vi "Get Server DLL Path.vi"() -> (0 "server dll path":path)   [LabVIEW 2019, in "grpc-lvsupport.lvlib"]
uses:
  grpc-lvsupport.lvlib
  <vilib>/Utility/LVLibp/NI_PackedLibraryUtility.lvlib
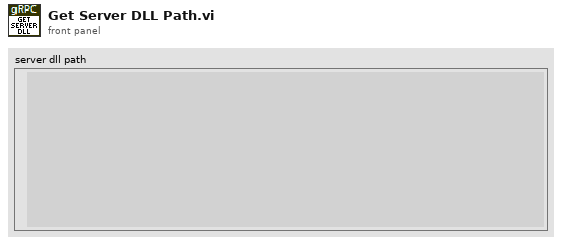
[diagram p1: front panel]
types:
  T1 = enum32{"invalid app kind", "Development System", "Run Time System", "Student Edition", "Embedded LabVIEW", "Evaluation", "Custom"}
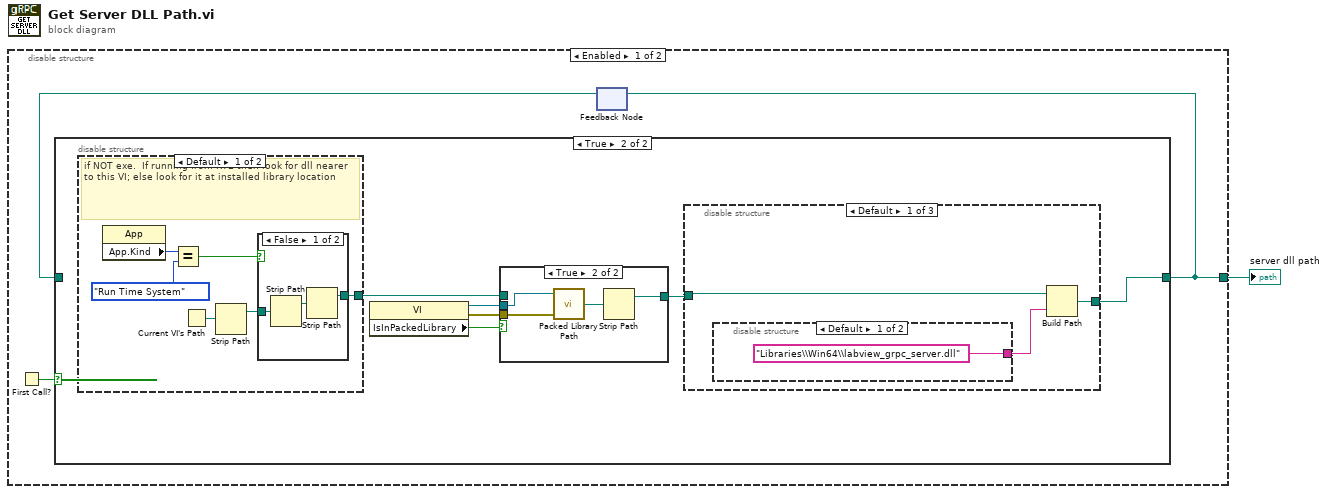
[diagram p0: block diagram]
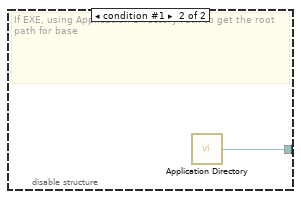
[diagram p5: hidden frame]
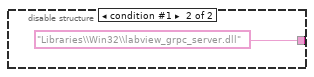
[diagram p6: hidden frame]
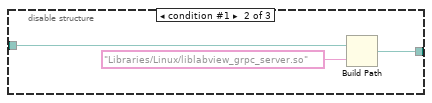
[diagram p7: hidden frame]
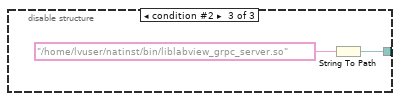
[diagram p8: hidden frame]
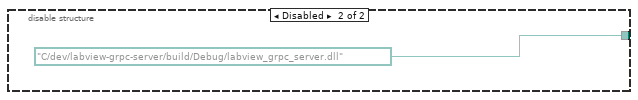
[diagram p9: hidden frame]
diagram:
  n1 = disable-structure shown="Enabled" {
    disable-tunnel: [w3 path "C:/dev/labview-grpc-server/build/Debug/labview_grpc_server.dll" ("Server dll path")] -> w1
    frame Enabled {
      n2 = First Call?() -> (First Call?: T/F=w4:bool)
      n3 = feedback #1() -> (w2:path)  [unwired: 1 in]
      n4 = case shown="True" w4 {
        tunnel: [w5 w6] -> w3
        tunnel: w2 -> [w5 _]
        frame False {
        }
        frame True {
          n5 = disable-structure shown="Default" {
            disable-tunnel: [w20 w27] -> w8
            frame condition #0 (active) {
              # "if NOT exe.  If running from RTE then look for dll nearer to this VI; else look for it at installed library location"
              n6 = property class="App"() -> ("App.Kind"=w19:T1)  [unwired: 2 in, 2 out]
              n7 = Equal?(x=w19, y=T1."Run Time System") -> (x = y?=w17:bool)
              n8 = Current VI's Path() -> (path=w21:path)
              n9 = Strip Path(path=w21) -> (stripped path=w22:path)  [unwired: 1 out]
              n10 = case shown="False" w17 {
                tunnel: w22 -> [w25 w26]
                tunnel: [w23 w26] -> w20
                frame False {
                  n11 = Strip Path(path=w25) -> (stripped path=w24:path)  [unwired: 1 out]
                  n12 = Strip Path(path=w24) -> (stripped path=w23:path)  [unwired: 1 out]
                }
                frame True {
                }
              }
            }
            frame condition #1 {
              # "If EXE, using Application Directory Path to get the root path for base"
              n13 = call <vilib>:"Application Directory.vi"() -> ("Application Directory"=w27:path)
            }
          }
          n14 = property class="VI"() -> (reference out=w10:refnum<vi>, error out=w11:errorcluster, "IsInPackedLibrary"=w9:bool)  [unwired: 2 in]
          n15 = case shown="True" w9 {
            tunnel: w10 -> [_ w16]
            tunnel: w11 -> [_ w15]
            tunnel: [w12 w14] -> w7
            tunnel: w8 -> [w12 _]
            frame False {
            }
            frame True {
              n16 = call <vilib>:"Packed Library Path.vi"("error in (no error)"=w15, "vi reference"=w16) -> ("packed library path"=w13:path)  [unwired: 1 in, 2 out]
              n17 = Strip Path(path=w13) -> (stripped path=w14:path)  [unwired: 1 out]
            }
          }
          n18 = disable-structure shown="Default" {
            disable-tunnel: w7 -> [w28 w35 _]
            disable-tunnel: [w29 w34 w36] -> w6
            frame condition #0 (active) {
              n19 = disable-structure shown="Default" {
                disable-tunnel: ["Libraries\\Win64\\labview_grpc_server.dll" ("name or relative path") "Libraries\\Win32\\labview_grpc_server.dll" ("name or relative path")] -> w30
                frame condition #0 (active) {
                }
                frame condition #1 {
                }
              }
              n20 = Build Path(base path=w28, name or relative path=w30) -> (appended path=w29:path)
            }
            frame condition #1 {
              n21 = Build Path(base path=w35, name or relative path="Libraries/Linux/liblabview_grpc_server.so") -> (appended path=w34:path)
            }
            frame condition #2 {
              n22 = String To Path(string="/home/lvuser/natinst/bin/liblabview_grpc_server.so" ("name or relative path")) -> (path=w36:path)
            }
          }
        }
      }
      n23 = feedback-in #1(w3) -> ()
    }
    frame Disabled {
    }
  }
  "server dll path" <- w1
